vi "sweep_voltage_measure_current.vi"() -> ()   [LabVIEW 2024]
uses:
  <vilib>/Analysis/1siggen.llb/Ramp Pattern by Delta.vi
  <vilib>/Utility/file.llb/Write Delimited Spreadsheet (string).vi
  <vilib>/Utility/file.llb/Write Delimited Spreadsheet (DBL).vi
  <vilib>/Analysis/NI_AALBase.lvlib
  Keithley_2450_2470_1_4_0_LV2015_NewReadme2_2450-LV2015-1.4.0/Keithley 2450/Keithley 2450.lvlib
panel:
  in  "time to wait between voltages":i32
  in  "Time to wait before current meas (ms)":i32
  out "Actual Voltage":dbl
  in  "Num Current Meas":i32=6
  in  "Path":path
  out "error out":errorcluster
  in  "error in (no error)":errorcluster
  in  "VISA resource name":refnum<visa-resource-name>
  out "Set Voltage":dbl
  in  "Step Size (V)":dbl=0.1 format="%#_13g"
  in  "Max V":dbl format="%#_13g"
  in  "Start V":dbl format="%#_13g"
  out "current":dbl
  in  "measurement interval":i32=200
  in  "Source Limit Level (0.1)":dbl=5e-08
  # "as of now it only records every 1V"
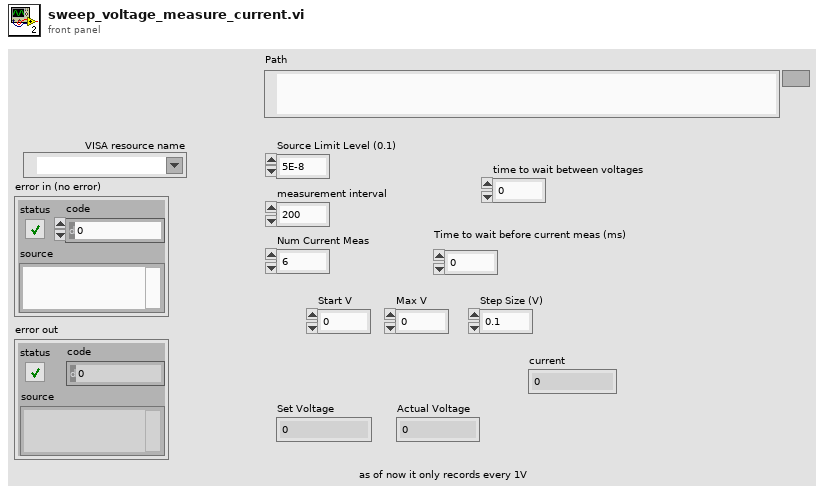
[diagram p1: front panel]
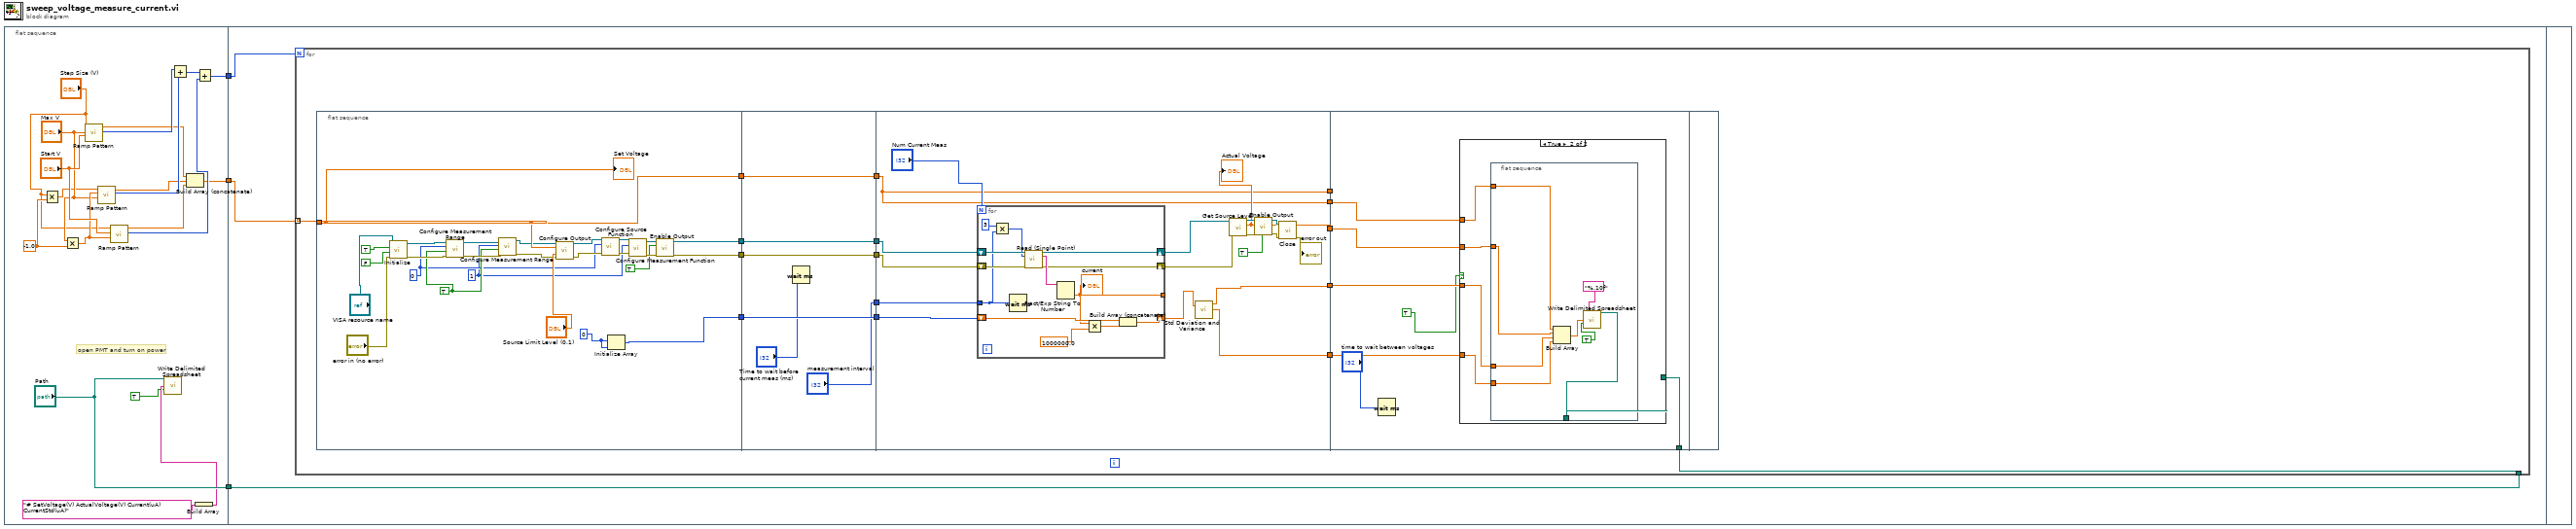
[diagram p0: block diagram]
diagram:
  n1 = flat-sequence {
    tunnel: [w12] -> w3
    tunnel: [w11] -> w2
    tunnel: ["Path"] -> w1
    tunnel: w3 -> [w25]
    tunnel: w2 -> [w24]
    tunnel: w1 -> [w23]
    frame #0 {
      w6 = -1.0
      # "open PMT and turn on power"
      n2 = Multiply(x="Step Size (V)", y=w6) -> (x*y=w4:dbl)
      n3 = Multiply(x="Max V", y=w6) -> (x*y=w14:dbl)
      n4 = call-poly <vilib>:"Ramp Pattern.vi"("start"="Start V", "end"="Max V", "delta"="Step Size (V)") -> ("samples"=w19:i32, "Ramp Pattern"=w16:dbl[])  [unwired: 6 in, 1 out]
      n5 = call-poly <vilib>:"Ramp Pattern.vi"("start"="Max V", "end"=w14, "delta"=w4) -> ("samples"=w20:i32, "Ramp Pattern"=w17:dbl[])  [unwired: 6 in, 1 out]
      n6 = call-poly <vilib>:"Ramp Pattern.vi"("start"=w14, "end"="Start V", "delta"="Step Size (V)") -> ("samples"=w22:i32, "Ramp Pattern"=w18:dbl[])  [unwired: 6 in, 1 out]
      n7 = Add(x=w19, y=w20) -> (x+y=w21:i32)
      n8 = Build Array (concatenate)(w16, w17, w18) -> (w12:dbl[])
      n9 = Build Array("# SetVoltage(V) ActualVoltage(V) Current(uA) CurrentStd(uA)") -> (w8:string[])
      n10 = call-poly <vilib>:"Write Delimited Spreadsheet.vi"("file path (dialog if empty)"="Path", "1D data"=w8, "append to file? (new file:F)"=TRUE) -> ()  [unwired: 11 in, 2 out]
      n11 = Add(x=w21, y=w22) -> (x+y=w11:i32)
    }
    frame #1 {
      n12 = for {
        N: w24 -> [_]
        tunnel: w25 -> [w41] mode=indexing
        tunnel: w23 -> [w40]
        n13 = flat-sequence {
          tunnel: w41 -> [w67]
          tunnel: [w67] -> w35
          tunnel: [w44] -> w32
          tunnel: [w43] -> w30
          tunnel: [w42] -> w28
          tunnel: w35 -> [w73]
          tunnel: [w73] -> w34
          tunnel: ["measurement interval"] -> w33
          tunnel: w32 -> [w72]
          tunnel: [w72] -> w31
          tunnel: w30 -> [w71]
          tunnel: [w71] -> w29
          tunnel: w28 -> [w70]
          tunnel: [w70] -> w27
          tunnel: [w81] -> w39
          tunnel: [w82] -> w38
          tunnel: [w76] -> w37
          tunnel: [w81] -> w36
          tunnel: w34 -> [w81]
          tunnel: w33 -> [w80]
          tunnel: w31 -> [w79]
          tunnel: w29 -> [w78]
          tunnel: w27 -> [w77]
          tunnel: [w74] -> w26
          tunnel: w40 -> [w111]
          tunnel: w39 -> [w110]
          tunnel: w38 -> [w109]
          tunnel: w37 -> [w108]
          tunnel: w36 -> [_]
          tunnel: w26 -> [w107]
          frame #0 {
            w51 = 0
            w50 = TRUE
            w47 = 1
            w49 = 0
            n14 = call "Initialize.vi"("error in (no error)"="error in (no error)", "Reset (True)"=FALSE, "ID Query (True)"=TRUE, "VISA resource name"="VISA resource name") -> ("error out"=w64:errorcluster, "VISA resource name out"=w65:refnum<visa-resource-name>)  [unwired: 6 in]
            n15 = call "Configure Measurement Range.vi"("error in (no error)"=w64, "Enable Auto Range (T:Enable)"=w50, "Function (0: Volts)"=w49, "VISA resource name"=w65) -> ("error out"=w63:errorcluster, "VISA resource name out"=w62:refnum<visa-resource-name>)  [unwired: 6 in]
            n16 = call "Configure Measurement Range.vi"("error in (no error)"=w63, "Enable Auto Range (T:Enable)"=w50, "Function (0: Volts)"=w47, "VISA resource name"=w62) -> ("error out"=w58:errorcluster, "VISA resource name out"=w54:refnum<visa-resource-name>)  [unwired: 6 in]
            n17 = call "Configure Output.vi"("VISA resource name"=w54, "Source Level (0)"=w67, "Source Limit Level (0.1)"="Source Limit Level (0.1)", "error in (no error)"=w58) -> ("VISA resource name out"=w55:refnum<visa-resource-name>, "error out"=w59:errorcluster)  [unwired: 10 in]
            n18 = call "Configure Source Function.vi"("error in (no error)"=w59, "Function (0: Volts)"=w49, "VISA resource name"=w55) -> ("error out"=w60:errorcluster, "VISA resource name out"=w56:refnum<visa-resource-name>)  [unwired: 7 in]
            n19 = Initialize Array(w51, w51) -> (w44:i32[])
            n20 = call "Configure Measurement Function.vi"("error in (no error)"=w60, "Function (0: Volts)"=w47, "VISA resource name"=w56) -> ("error out"=w61:errorcluster, "VISA resource name out"=w57:refnum<visa-resource-name>)  [unwired: 7 in]
            n21 = call "Enable Output.vi"("error in (no error)"=w61, "Enable Output (T: Enable)"=TRUE, "VISA resource name"=w57) -> ("error out"=w43:errorcluster, "VISA resource name out"=w42:refnum<visa-resource-name>)  [unwired: 7 in]
            "Set Voltage" <- w67
          }
          frame #1 {
            n22 = Wait (ms)(milliseconds to wait="Time to wait before current meas (ms)") -> ()  [unwired: 1 out]
          }
          frame #2 {
            n23 = for {
              N: "Num Current Meas" -> [_]
              tunnel: [w93] -> _
              shift-right: [w103] -> w88
              shift-left: w78 -> [w102]
              shift-right: [w101] -> w91
              shift-left: w77 -> [w100]
              tunnel: w80 -> [w97]
              shift-right: [w95] -> w75
              shift-left: w79 -> [w96]
              n24 = Multiply(x=3, y=w97) -> (x*y=w99:i32)
              n25 = Wait (ms)(milliseconds to wait=w97) -> ()  [unwired: 1 out]
              n26 = call "Read (Single Point).vi"("VISA resource name"=w100, "Timeout (10000 ms)"=w99, "error in (no error)"=w102) -> ("VISA resource name out"=w101:refnum<visa-resource-name>, "Data out"=w104:string, "error out"=w103:errorcluster)  [unwired: 10 in]
              n27 = Fract/Exp String To Number(string=w104) -> (number=w93:dbl)  [unwired: 3 in, 1 out]
              "current" <- w93
              n28 = Multiply(x=w93, y=1000000.0) -> (x*y=w92:dbl)
              n29 = Build Array (concatenate)(w96, w92) -> (w95:dbl[])
            }
            n30 = call <vilib>:"Std Deviation and Variance.vi"("X"=w75) -> ("mean"=w76:dbl, "standard deviation"=w74:dbl)  [unwired: 1 in, 1 out]
            n31 = call "Get Source Level.vi"("error in (no error)"=w88, "VISA resource name"=w91) -> ("error out"=w89:errorcluster, "Voltage Level Out"=w82:dbl, "VISA resource name out"=w90:refnum<visa-resource-name>)  [unwired: 6 in, 1 out]
            "Actual Voltage" <- w82
            n32 = call "Enable Output.vi"("error in (no error)"=w89, "Enable Output (T: Enable)"=TRUE, "VISA resource name"=w90) -> ("error out"=w84:errorcluster, "VISA resource name out"=w85:refnum<visa-resource-name>)  [unwired: 7 in]
            n33 = call "Close.vi"("error in (no error)"=w84, "VISA resource name"=w85) -> ("error out"=→"error out":errorcluster)  [unwired: 9 in]
          }
          frame #3 {
            n34 = Wait (ms)(milliseconds to wait="time to wait between voltages") -> ()  [unwired: 1 out]
            n35 = case shown="True" TRUE {
              tunnel: w111 -> [_ w116]
              tunnel: w110 -> [_ w115]
              tunnel: w109 -> [_ w114]
              tunnel: w108 -> [_ w113]
              tunnel: w107 -> [_ w112]
              frame False {
              }
              frame True {
                n36 = flat-sequence {
                  tunnel: w116 -> [w124]
                  tunnel: w115 -> [w120]
                  tunnel: w113 -> [w118]
                  tunnel: w114 -> [w119]
                  tunnel: w112 -> [w117]
                  frame #0 {
                    n37 = Build Array(w120, w119, w118, w117) -> (w123:dbl[])
                    n38 = call-poly <vilib>:"Write Delimited Spreadsheet.vi"("file path (dialog if empty)"=w124, "format (%.3f)"="%.10f", "1D data"=w123, "append to file? (new file:F)"=TRUE) -> ()  [unwired: 10 in, 2 out]
                  }
                }
              }
            }
          }
          frame #4 {
          }
        }
      }
    }
    frame #2 {
    }
  }
